vi "multply.vi"() -> ()   [LabVIEW 2020]
panel:
  in  "Library Path":path=path "/home/saman/src/lvcc/build/test/libtest.so"
  in  "a":i32=3
  in  "b":i32=2
  out "return type":i32
  out "error out":errorcluster
  # "x"
  # "="
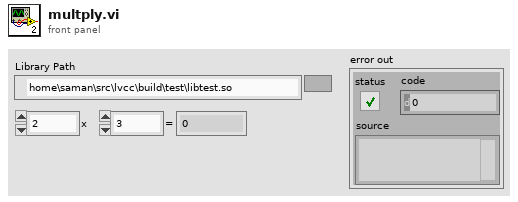
[diagram p1: front panel]
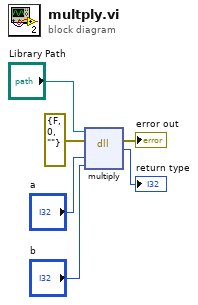
[diagram p0: block diagram]
diagram:
  n1 = dll-call lib="home/saman/src/lvcc/build/test/libtest.so" fn="multiply"(path in="Library Path", error in=errorcluster {"status"=FALSE, "code"=0, "source"=""} ("error in (no error)"), "a"="a", "b"="b") -> (error out=→"error out":errorcluster, "return type"=→"return type":i32)  [unwired: 3 in, 1 out]
